vi "DataPacker_SetMIDASAddress.vi"(8 "error in (no error)":errorcluster, 10 "Address to Log To":u32, 11 "DataPacker in":refnum<class "DataPacker.lvclass">) -> (0 "error out":errorcluster, 3 "DataPacker out":refnum<class "DataPacker.lvclass">)   [LabVIEW 2018, in "feGEM DataPacker.lvlib" / "DataPacker.lvclass"]
uses:
  DataPacker.lvclass
  DataPacker.lvclass/DataPacker.ctl
  <vilib>/Utility/SystemLogging/NI_SystemLogging.lvlib
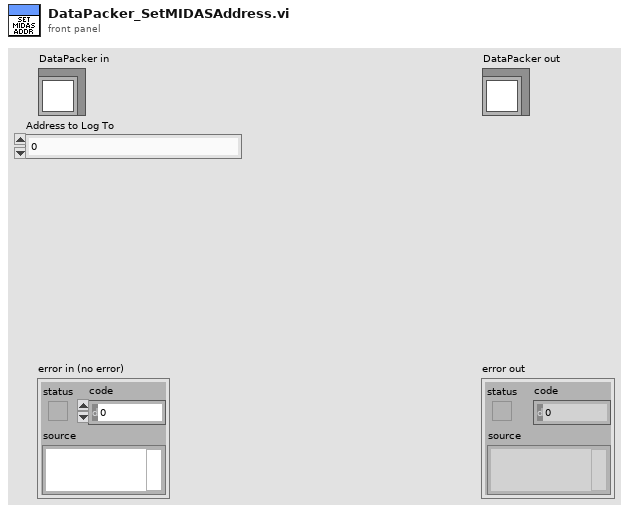
[diagram p1: front panel]
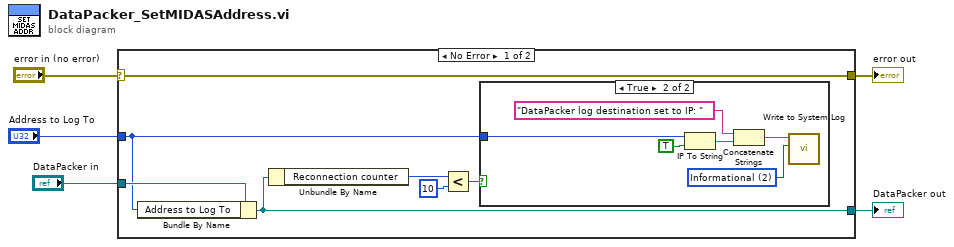
[diagram p0: block diagram]
diagram:
  n1 = case shown="No Error" "error in (no error)" {
    selector: "error in (no error)" -> [w12 w19]
    tunnel: [w12 w19] -> w4
    tunnel: [w9 w20] -> w2
    tunnel: "DataPacker in" -> [w11 w20]
    tunnel: "Address to Log To" -> [w10 _]
    frame No Error {
      n2 = Bundle By Name(cluster=w11, "Address to Log To"=w10) -> (w9:refnum<class "DataPacker.lvclass">)
      n3 = Unbundle By Name(w9) -> ("Reconnection counter"=w7:i32)
      n4 = Less?(x=w7, y=10) -> (x < y?=w6:bool)
      n5 = case shown="True" w6 {
        tunnel: w10 -> [_ w16]
        frame False {
        }
        frame True {
          w13 = 2 items=["Error", "Warning", "Informational"] ("severity")
          n6 = IP To String(1:TRUE ("dot notation? (F)"), 2:w16) -> (0:w17:string)
          n7 = Concatenate Strings("DataPacker log destination set to IP: " ("message"), w17) -> (w14:string)
          n8 = call <vilib>:"Write to System Log.vi"("severity"=w13, "message"=w14) -> ()  [unwired: 9 in, 1 out]
        }
      }
    }
    frame Error {
    }
  }
  "error out" <- w4
  "DataPacker out" <- w2
